vi "Search for App Source Folder.vi"(8 "error in":errorcluster) -> (0 "error out":errorcluster, 3 "App Source Path":path)   [LabVIEW 2020, in "hse-misc.lvlib"]
doc: "Search for the application source folder down the folder hierarchy, starting at the current project path. Finds the app source folder if it is in one of the folders down the hierarchy (e.g. when using the hse project structure).\n\n____\nHAMPEL SOFTWARE ENGINEERING v3.8.0 (2023-12-18 14:41)"
uses:
  hse-misc.lvlib
  <vilib>/regexp/Match Regular Expression.xnode
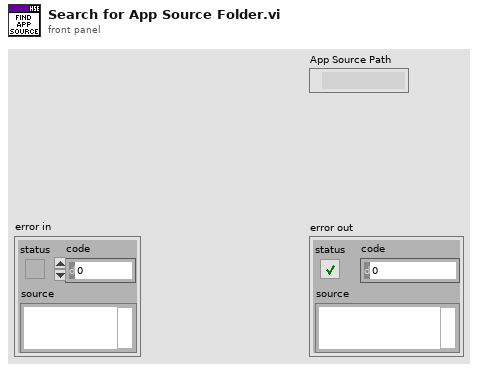
[diagram p1: front panel]
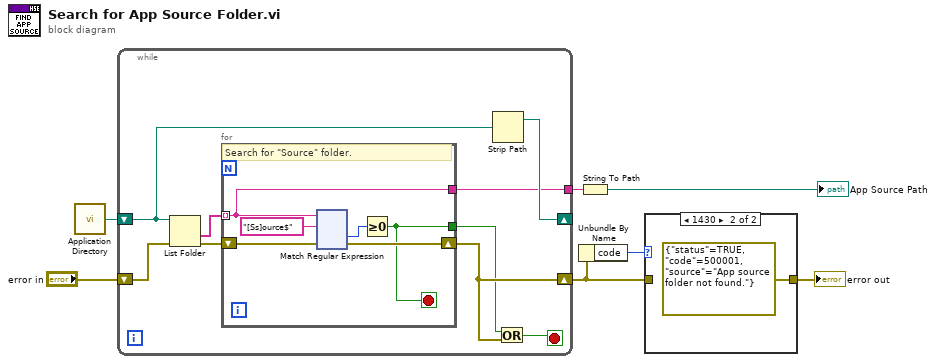
[diagram p0: block diagram]
diagram:
  n1 = call <vilib>:"Application Directory.vi"() -> ("Application Directory"=w7:path)
  n2 = while {
    shift-right: [w16] -> _
    shift-left: w7 -> [w9]
    shift-right: [w14] -> w3
    shift-left: "error in" -> [w11]
    tunnel: [w15] -> w5
    stop <- w12 stop-if-true
    n3 = List Folder(path=w9, error in=w11) -> (folder names=w8:string[], error out=w10:errorcluster)  [unwired: 2 in, 2 out]
    n4 = for {
      tunnel: w8 -> [w17] mode=indexing
      shift-right: [w19] -> w14
      shift-left: w10 -> [w22]
      tunnel: [w18] -> w13
      tunnel: [w17] -> w15
      stop <- w18 stop-if-true
      # "Search for \"Source\" folder."
      n5 = xnode "Match Regular Expression"("input string"=w17, "regular expression"="[Ss]ource$", "error in"=w22) -> ("offset past match"=w20:i32, "error out"=w19:errorcluster)  [unwired: 3 in, 3 out]
      n6 = Greater Or Equal To 0?(x=w20) -> (x >= 0?=w18:bool)
    }
    n7 = Strip Path(path=w9) -> (stripped path=w16:path)  [unwired: 1 out]
    n8 = Or(x=w13, y=w14) -> (x .or. y?=w12:bool)
  }
  n9 = Unbundle By Name(w3) -> ("code"=w2:i32)
  n10 = String To Path(string=w5) -> (path=→"App Source Path":path)
  n11 = case shown="1430" w2 {
    tunnel: w3 -> [w137 _]
    tunnel: [w137 errorcluster {"status"=TRUE, "code"=500001, "source"="App source folder not found."} ("error in")] -> w1
    frame 0, Default {
    }
    frame 1430 {
    }
  }
  "error out" <- w1
